vi "LABVIEW做的蓝牙数据发送程序.vi"() -> ()   [LabVIEW 2014]
panel:
  out "bytes written":i32
  in  "?":bool
  in  "数据输入":string
  in  "超时毫秒(60000)":i32
  in  "索引 2":i32
  out "设备清单":T1(array[cluster])
  out "service list":T2(array[cluster]) caption="服务列表"
  out "number of services":u16 caption="服务数量"
  out "address out":string caption="地址输出"
  in  "索引":i32
  out "设备数量":u16
  in  "时间限制ms(10000)":i32
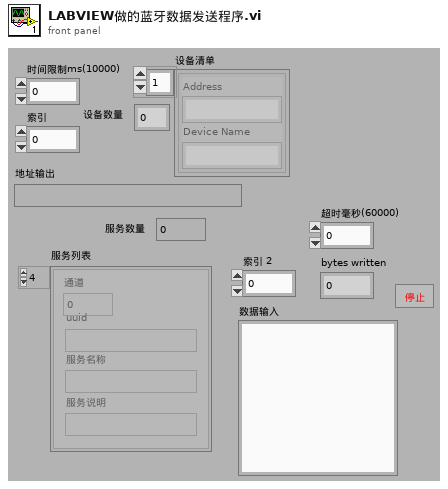
[diagram p1: front panel]
types:
  T1 = cluster{"Address":string, "Device Name":string}[]
  T2 = cluster{"channel":u16, "uuid":string, "service name":string, "service description":string}[]
  T3 = cluster{"channel":u16, "uuid":string, "service name":string, "service description":string}
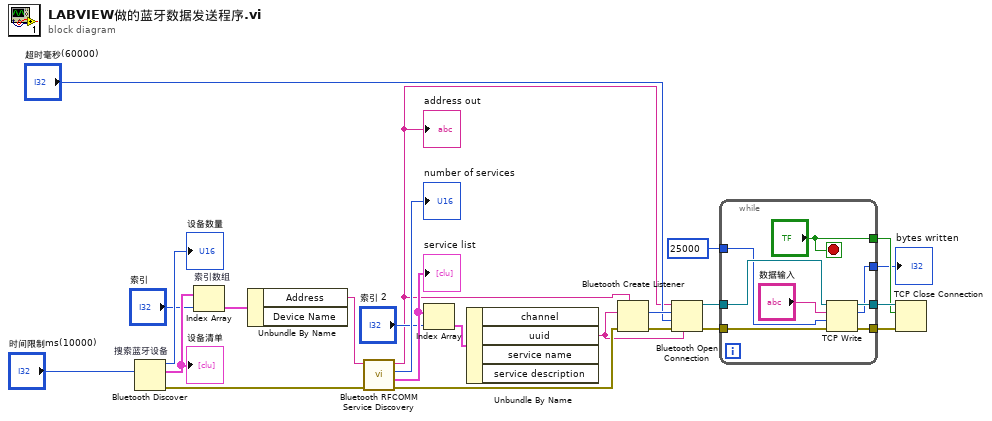
[diagram p0: block diagram]
diagram:
  n1 = Bluetooth Discover "搜索蓝牙设备"(10:"时间限制ms(10000)") -> (0:w9:errorcluster, 2:w22:T1, 3:→"设备数量":u16)  [unwired: 1 in]
  "设备清单" <- w22
  n2 = Index Array "索引数组"(array=w22, index="索引") -> (element=w20:cluster{"Address":string, "Device Name":string})
  n3 = Unbundle By Name(w20) -> ("Address"=w19:string)  [unwired: 1 out]
  n4 = call <vilib>:"Bluetooth RFCOMM Service Discovery.vi"("error in (no error)"=w9, "address in"=w19) -> ("error out"=w10:errorcluster, "service list"=w17:T2, "number of services"=→"number of services":u16, "address out"=w11:string)  [unwired: 2 in]
  "address out" <- w11
  "service list" <- w17
  n5 = Index Array(array=w17, index="索引 2") -> (element=w15:T3)
  n6 = Unbundle By Name(w15) -> ("uuid"=w5:string)  [unwired: 3 out]
  n7 = Bluetooth Create Listener(7:w11, 8:w10, 10:w5) -> (0:w14:errorcluster, 2:w13:u16)  [unwired: 1 in, 1 out]
  n8 = Bluetooth Open Connection(6:w5, 8:w14, 9:"超时毫秒(60000)", 10:w13, 11:w11) -> (0:w8:errorcluster, 3:w7:refnum<k31>)
  n9 = while {
    tunnel: w8 -> [w32]
    tunnel: w7 -> [w31]
    tunnel: 25000 ("超时毫秒(25000)") -> [w30]
    tunnel: [w28] -> w3
    tunnel: [w27] -> w1
    tunnel: [w26] -> w4
    tunnel: ["?"] -> w2
    stop <- "?" stop-if-true
    n10 = TCP Write(connection ID=w31, data in="数据输入", error in (no error)=w32, 9:w30) -> (connection ID out=w28:refnum<k31>, bytes written=w27:i32, error out=w26:errorcluster)
  }
  "bytes written" <- w1
  n11 = TCP Close Connection(connection ID=w3, abort (F)=w2, error in (no error)=w4) -> ()  [unwired: 2 out]
